vi "APSxStringToSensorBits.vi"(8 "error in (no error)":errorcluster caption="错误输入（无错误）", 9 "AutoDetect":i32, 10 "InitialBitString":string, 11 "hSENSOR":i32) -> (0 "error out":errorcluster caption="错误输出", 2 "Message":string, 3 "hSENSOR out":i32)   [LabVIEW 2018]
doc: "该模板用于创建子VI。"
uses:
  APSx.dll/APSx.dll
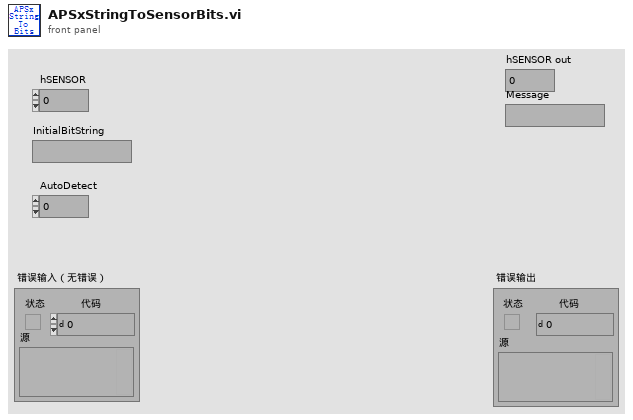
[diagram p1: front panel]
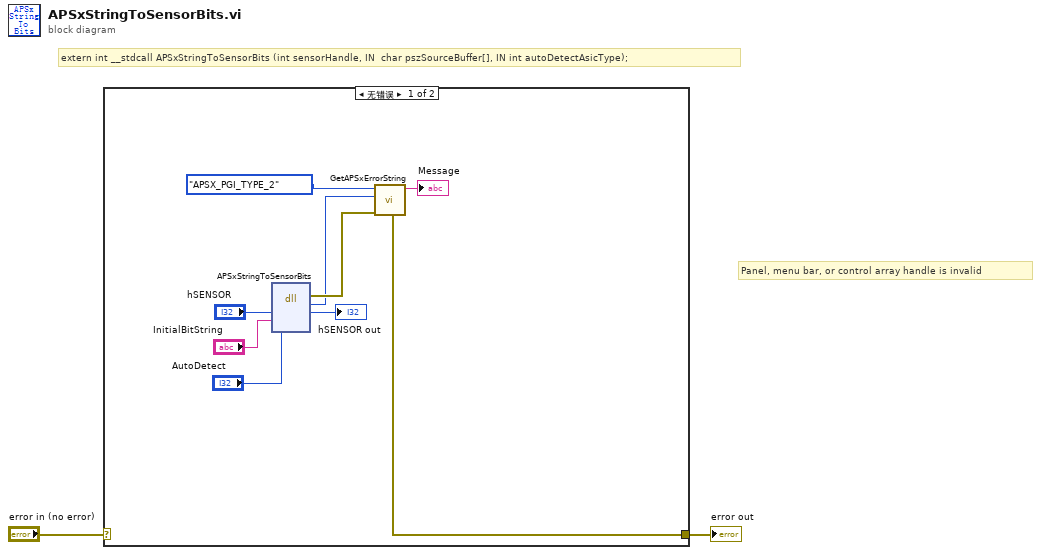
[diagram p0: block diagram]
diagram:
  # "Panel, menu bar, or control array handle is invalid"
  # "extern int __stdcall APSxStringToSensorBits (int sensorHandle, IN  char pszSourceBuffer[], IN int autoDetectAsicType);"
  n1 = case shown="无错误" "error in (no error)" {
    selector: "error in (no error)" -> [_ w12]
    tunnel: [w5 w12] -> w1
    frame No Error {
      n2 = dll-call lib="PTH2]abs D项目Feng恒隆项目Labview传感器对中台SourcesAPSx.dllAPSx.dll" fn="APSxStringToSensorBits"("hSENSOR"="hSENSOR", "InitialBitString"="InitialBitString", "AutoDetect"="AutoDetect") -> (error out=w7:errorcluster, "Code"=w6:i32, "hSENSOR"=→"hSENSOR out":i32)  [unwired: 5 in, 1 out]
      n3 = call "GetAPSxErrorString.vi"("error in (no error)"=w7, "ErrorCode"=w6, "PGIType"=enum16{"APSX_PGI_TYPE_1", "APSX_PGI_TYPE_2"}."APSX_PGI_TYPE_2") -> ("error out"=w5:errorcluster, "Message"=→"Message":string)  [unwired: 7 in]
    }
    frame Error {
    }
  }
  "error out" <- w1
